vi "Calibration Save.vi"(8 "error in (no error)":errorcluster, 11 "VISA resource name":refnum<visa-resource-name>="GPIB0::24::INSTR") -> (0 "error out":errorcluster, 3 "VISA resource name out":refnum<visa-resource-name>)   [LabVIEW 2018, in "Keithley 2450.lvlib"]
doc: "This VI saves calibration data to EEPROM."
uses:
  <instrlib>/Keithley 2450/Keithley 2450.lvlib
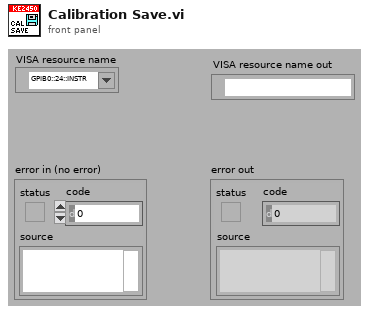
[diagram p1: front panel]
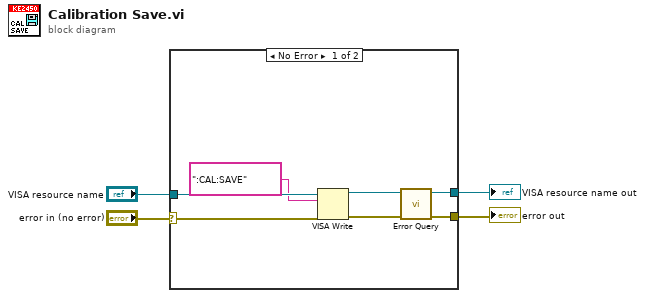
[diagram p0: block diagram]
diagram:
  n1 = case shown="No Error" "error in (no error)" {
    selector: "error in (no error)" -> [w11 w13]
    tunnel: [w8 w13] -> w3
    tunnel: "VISA resource name" -> [w10 w12]
    tunnel: [w5 w12] -> w1
    frame No Error {
      n2 = VISA Write(VISA resource name=w10, write buffer=":CAL:SAVE" ("string"), error in (no error)=w11) -> (VISA resource name out=w7:refnum<visa-resource-name>, error out=w6:errorcluster)  [unwired: 1 out]
      n3 = call <instrlib>:"Error Query.vi"("error in (no error)"=w6, "VISA resource name"=w7) -> ("error out"=w8:errorcluster, "VISA resource name out"=w5:refnum<visa-resource-name>)  [unwired: 6 in, 2 out]
    }
    frame Error {
      # "Do nothing if error condition"
    }
  }
  "error out" <- w3
  "VISA resource name out" <- w1
